vi "Emballage_GVF_Chemin_Son.vi"(8 "entrée d'erreur (pas d'erreur)":errorcluster, 11 "Énum":enum16{"get", "set"}(ring)) -> (0 "sortie d'erreur":errorcluster, 1 "Chemin lazer.WAV":path, 2 "Chemin Utopia - Question.WAV":path, 3 "Chemin The Microsoft Sound.wav":path, 5 "Chemin Utopia - Erreur.WAV":path)   [LabVIEW 2020]
uses:
  Modules/FS/60_FS_Controles/60_FS_SetGet.ctl
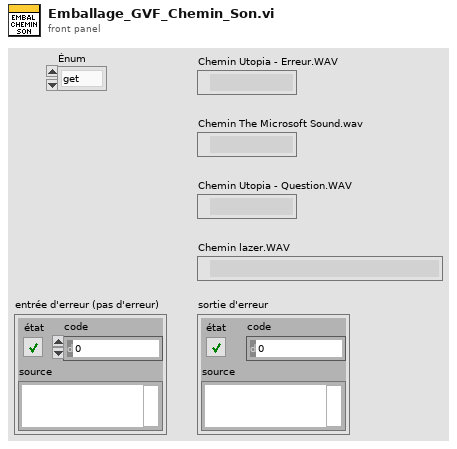
[diagram p1: front panel]
types:
  T1 = typedef "60_FS_SetGet.ctl" = enum16{"set", "get"}
  T2 = cluster{"Admin-réseau":path, "XML-Réseau":path, " Résultat tests-Réseau":path, " Archive prôbleme-Réseau":path, " Archive Test  Local":path}
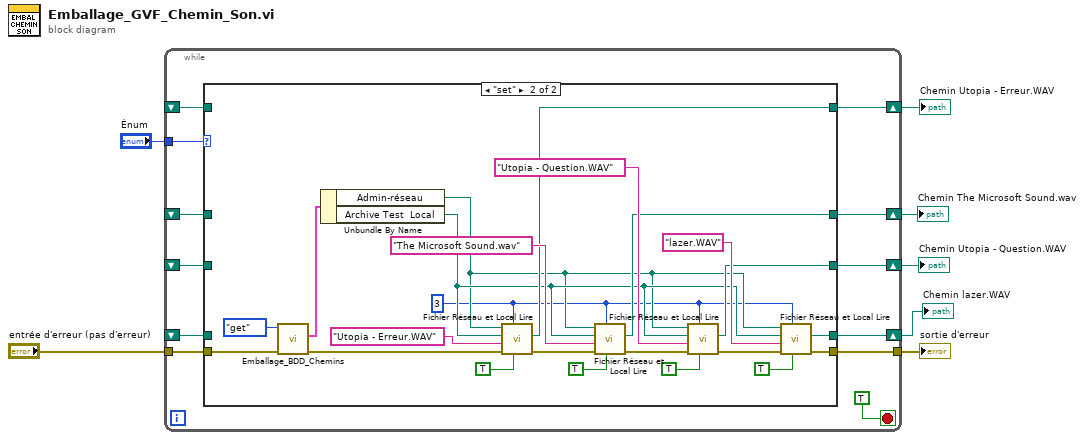
[diagram p0: block diagram]
diagram:
  n1 = while {
    tunnel: "Énum" -> [w18]
    shift-right: [w14] -> w3
    shift-left: _ -> [w13]
    shift-right: [w16] -> w5
    shift-left: _ -> [w11]
    shift-right: [w17] -> w6
    shift-left: _ -> [w10]
    shift-right: [w15] -> w4
    shift-left: _ -> [w12]
    tunnel: "entrée d'erreur (pas d'erreur)" -> [w9]
    tunnel: [w8] -> w2
    stop <- TRUE stop-if-true
    n2 = case shown="\"set\"" w18 {
      tunnel: [w21 w36] -> w17
      tunnel: [w22 w35] -> w16
      tunnel: [w23 w34] -> w15
      tunnel: [w24 w33] -> w14
      tunnel: w13 -> [w24 _]
      tunnel: w12 -> [w23 _]
      tunnel: w11 -> [w22 _]
      tunnel: w10 -> [w21 _]
      tunnel: w9 -> [w20 w31]
      tunnel: [w20 w32] -> w8
      frame "get", Default {
      }
      frame "set" {
        w25 = 3 ("nbr de sous dossier")
        n3 = call "Emballage_BDD_Chemins.vi"("error in (no error)"=w31, "SetGet"=60_FS_SetGet."get") -> ("error out"=w30:errorcluster, "CLT_Chemins_out"=w29:T2)  [unwired: 8 in]
        n4 = Unbundle By Name(w29) -> ("Admin-réseau"=w26:path, "Archive Test  Local"=w27:path)
        n5 = call "Fichier Réseau et Local Lire .vi"("reseau prioritaire ?"=TRUE, "nbr de sous dossier"=w25, "error in"=w30, "Nom fichier"="Utopia - Erreur.WAV", "Dossier Local"=w27, "Fichier ou dossier Reseau"=w26) -> ("error out"=w45:errorcluster, "Chemin OUT"=w33:path)  [unwired: 1 in, 2 out]
        n6 = call "Fichier Réseau et Local Lire .vi"("reseau prioritaire ?"=TRUE, "nbr de sous dossier"=w25, "error in"=w45, "Nom fichier"="The Microsoft Sound.wav", "Dossier Local"=w27, "Fichier ou dossier Reseau"=w26) -> ("error out"=w46:errorcluster, "Chemin OUT"=w34:path)  [unwired: 1 in, 2 out]
        n7 = call "Fichier Réseau et Local Lire .vi"("reseau prioritaire ?"=TRUE, "nbr de sous dossier"=w25, "error in"=w46, "Nom fichier"="Utopia - Question.WAV", "Dossier Local"=w27, "Fichier ou dossier Reseau"=w26) -> ("error out"=w47:errorcluster, "Chemin OUT"=w35:path)  [unwired: 1 in, 2 out]
        n8 = call "Fichier Réseau et Local Lire .vi"("reseau prioritaire ?"=TRUE, "nbr de sous dossier"=w25, "error in"=w47, "Nom fichier"="lazer.WAV", "Dossier Local"=w27, "Fichier ou dossier Reseau"=w26) -> ("error out"=w32:errorcluster, "Chemin OUT"=w36:path)  [unwired: 1 in, 2 out]
      }
    }
  }
  "Chemin lazer.WAV" <- w6
  "Chemin Utopia - Question.WAV" <- w5
  "Chemin The Microsoft Sound.wav" <- w4
  "Chemin Utopia - Erreur.WAV" <- w3
  "sortie d'erreur" <- w2
